vi "initRIOConfig.vi"(8 "error in (no error)":errorcluster, 11 "RIOConfig in":refnum<class "RIOConfig.lvclass">) -> (0 "error out":errorcluster, 3 "RIOConfig out":refnum<class "RIOConfig.lvclass">)   [LabVIEW 2013, in "ComponentData.lvlib" / "RIOConfig.lvclass"]
uses:
  <userlib>/Common/Component/Application/RT/ComponentData/ConfigurationHandler/RIOConfig/RIOConfig.lvclass
  <userlib>/Common/Component/Application/MyComputer/ComponentConfiguration/ComponentConfigurationTypedefs/rioConfig.ctl
  <userlib>/Common/Component/Application/RT/ComponentData/ConfigurationHandler/RIOConfig/RIOConfig.lvclass/RIOConfig.ctl
  <vilib>/Utility/xml.llb/Read From XML File(string).vi
  <userlib>/Common/Component/Application/MyComputer/ComponentConfiguration.lvlib
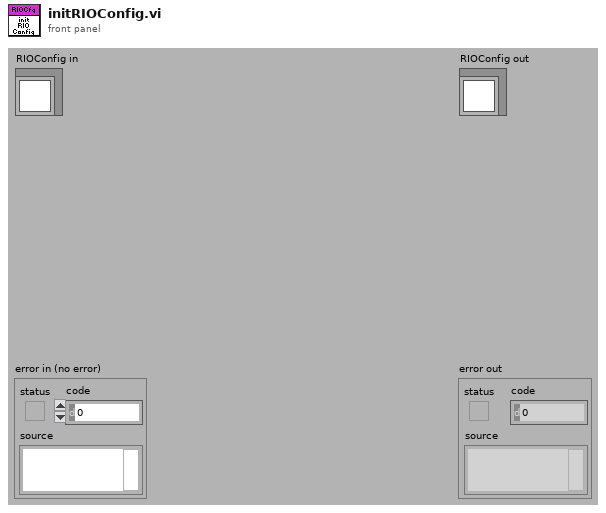
[diagram p1: front panel]
types:
  T1 = typedef "ComponentConfiguration.lvlib/rioConfig.ctl" = cluster{"rioResourceName":string}
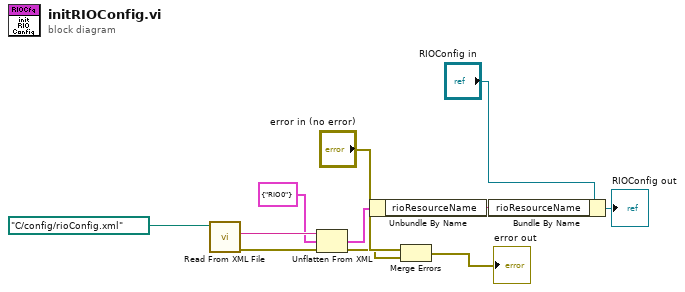
[diagram p0: block diagram]
diagram:
  n1 = call-poly <vilib>:"Read From XML File.vi"("XML File Path"=path "C:/config/rioConfig.xml" ("configuration file path")) -> ("error out"=w4:errorcluster, "XML Elements"=w8:string)  [unwired: 8 in, 1 out]
  n2 = Unflatten From XML(xml string=w8, type=T1 {"rioResourceName"="RIO0"} ("rioConfig"), error in (no error)=w4) -> (value=w6:T1, error out=w2:errorcluster)
  n3 = Unbundle By Name(w6) -> ("rioResourceName"=w5:string)
  n4 = Merge Errors("error in (no error)", w2) -> (→"error out":errorcluster)
  n5 = Bundle By Name(cluster="RIOConfig in", "rioResourceName"=w5) -> (→"RIOConfig out":refnum<class "RIOConfig.lvclass">)
